vi "Traegergas ermitteln Ring Index.vi"(8 "error in (no error)":errorcluster caption="Fehler (Eingang, kein Fehler)", 10 "Trägergas":T1 caption="Carrier Gas", 11 "Ring (Eingang)":refnum<vi>) -> (0 "error out":errorcluster caption="Fehler (Ausgang)", 2 "found":bool, 3 "Ring Index":i32)   [LabVIEW 2020, in "System Einstellungen V2.lvlib"]
uses:
  System Einstellungen V2.lvlib
  Traegergas.ctl
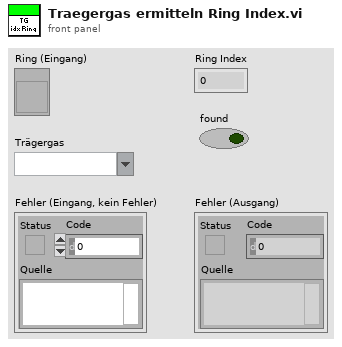
[diagram p1: front panel]
types:
  T1 = typedef "System Einstellungen V2.lvlib/Traegergas.ctl" = string
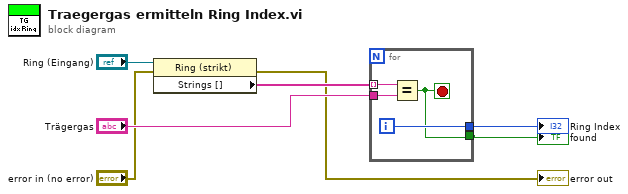
[diagram p0: block diagram]
diagram:
  n1 = property class="Ring (strikt)"(reference="Ring (Eingang)", error in="error in (no error)") -> (error out=→"error out":errorcluster, "Strings []"=w6:string[])  [unwired: 1 out]
  n2 = for {
    tunnel: w6 -> [w11] mode=indexing
    tunnel: "Trägergas" -> [w10]
    tunnel: [w9] -> w7
    tunnel: [w8] -> w1
    i -> [w9]
    stop <- w8 stop-if-true
    n3 = Equal?(x=w11, y=w10) -> (x = y?=w8:bool)
  }
  "Ring Index" <- w7
  "found" <- w1
